vi "Freetype Error.vi"(8 "error in (no error)":errorcluster, 11 "Error":i32) -> (0 "error out":errorcluster)   [LabVIEW 2023, in "Freetype Drawer.lvlib"]
uses:
  Freetype Drawer.lvlib
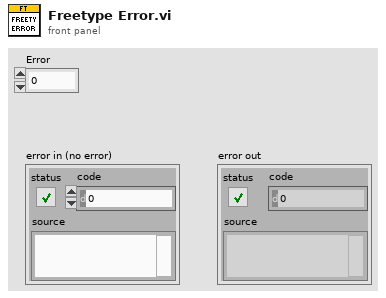
[diagram p1: front panel]
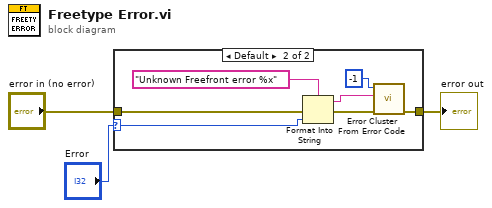
[diagram p0: block diagram]
diagram:
  n1 = case shown="Default" "Error" {
    selector: "Error" -> [_ w5]
    tunnel: "error in (no error)" -> [w4 w11]
    tunnel: [w4 w10] -> w1
    frame 0 {
    }
    frame Default {
      n2 = Format Into String(format string="Unknown Freefront error %x" ("error message (\"\")"), error in=w11, w5) -> (resulting string=w7:string, error out=w8:errorcluster)  [unwired: 1 in]
      n3 = call <vilib>:"Error Cluster From Error Code.vi"("error in (no error)"=w8, "error message (\"\")"=w7, "error code (0)"=-1) -> ("error out"=w10:errorcluster)  [unwired: 6 in]
    }
  }
  "error out" <- w1
